vi "Flame Detect Debug.vi"() -> ()   [LabVIEW 2013]
panel:
  in  "Board":enum16{"Rows 1-8", "Rows 9-17", "Rows 18-24"}(ring)
  out "Waveform Chart":T1(graph)
  in  "stop":bool
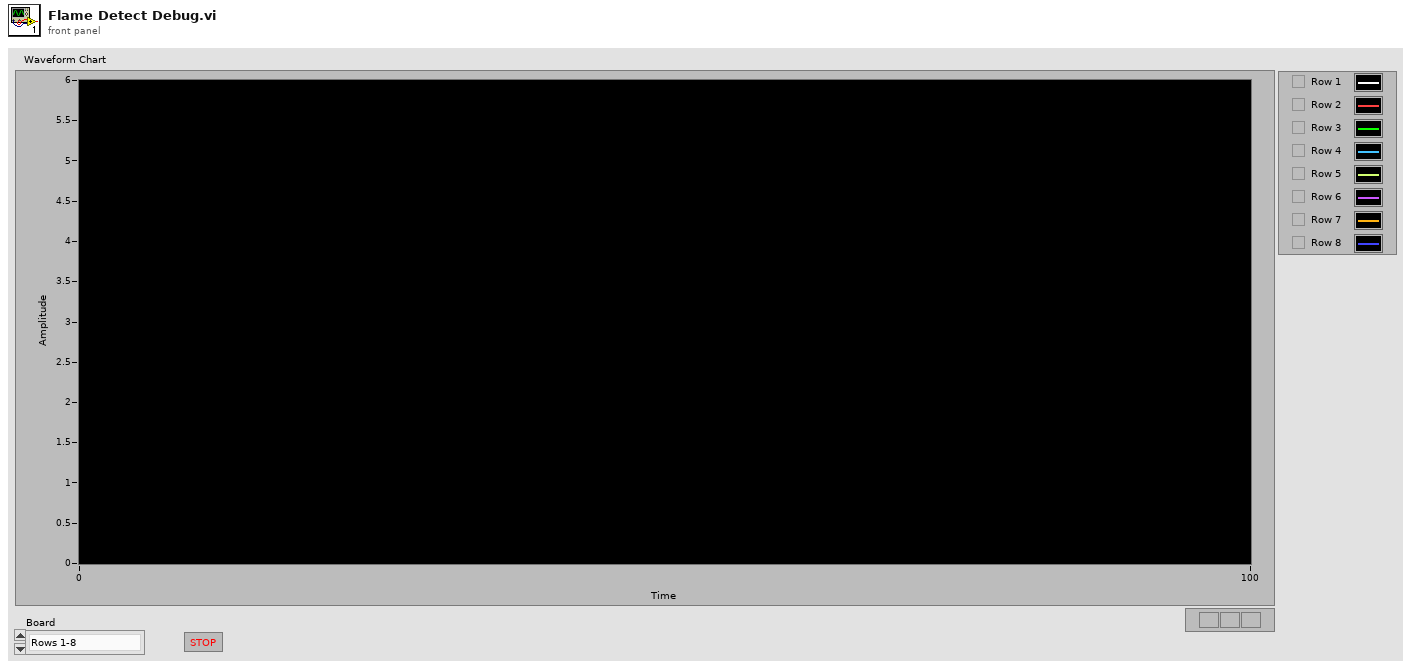
[diagram p1: front panel]
types:
  T1 = cluster{"[0]":dbl, "[1]":dbl, "[2]":dbl, "[3]":dbl, "[4]":dbl, "[5]":dbl, "[6]":dbl, "[7]":dbl, "[8]":dbl}
  T2 = enum16{"HSCAN", "MSCAN", "SWCAN", "LSFTCAN", "HSCAN2", "HSCAN3"}
  T3 = cluster{"DeviceType":i32, "Handle":i32, "NumberOfClients":i32, "SerialNumber":i32, "MaxAllowedClients":i32}[]
  T4 = cluster{"DeviceType":i32, "Handle":i32, "NumberOfClients":i32, "SerialNumber":i32, "MaxAllowedClients":i32}
  T5 = typedef "ctl spymessage.ctl" = cluster{"StatusBitField":u32, "StatusBitField2":u32, "TimeHardware":u32, "TimeHardware2":u32, "TimeSystem":u32, "TimeSystem2":u32, "TimeStampHardwareID":u8, "TimeStampHardwareID2":u8, "NetworkID":u8, "NodeID":u8, "Protocol":u8, "MessagePieceID":u8, "ColorID":u8, "NumberBytesHeader":u8, "NumberBytesData":u8, "DescriptionID":u16, "ArbIDOrHeader":u32, "Data [8]":u8[], "AckBytes [8]":u8[], "Value":sgl, "MiscData":u8}
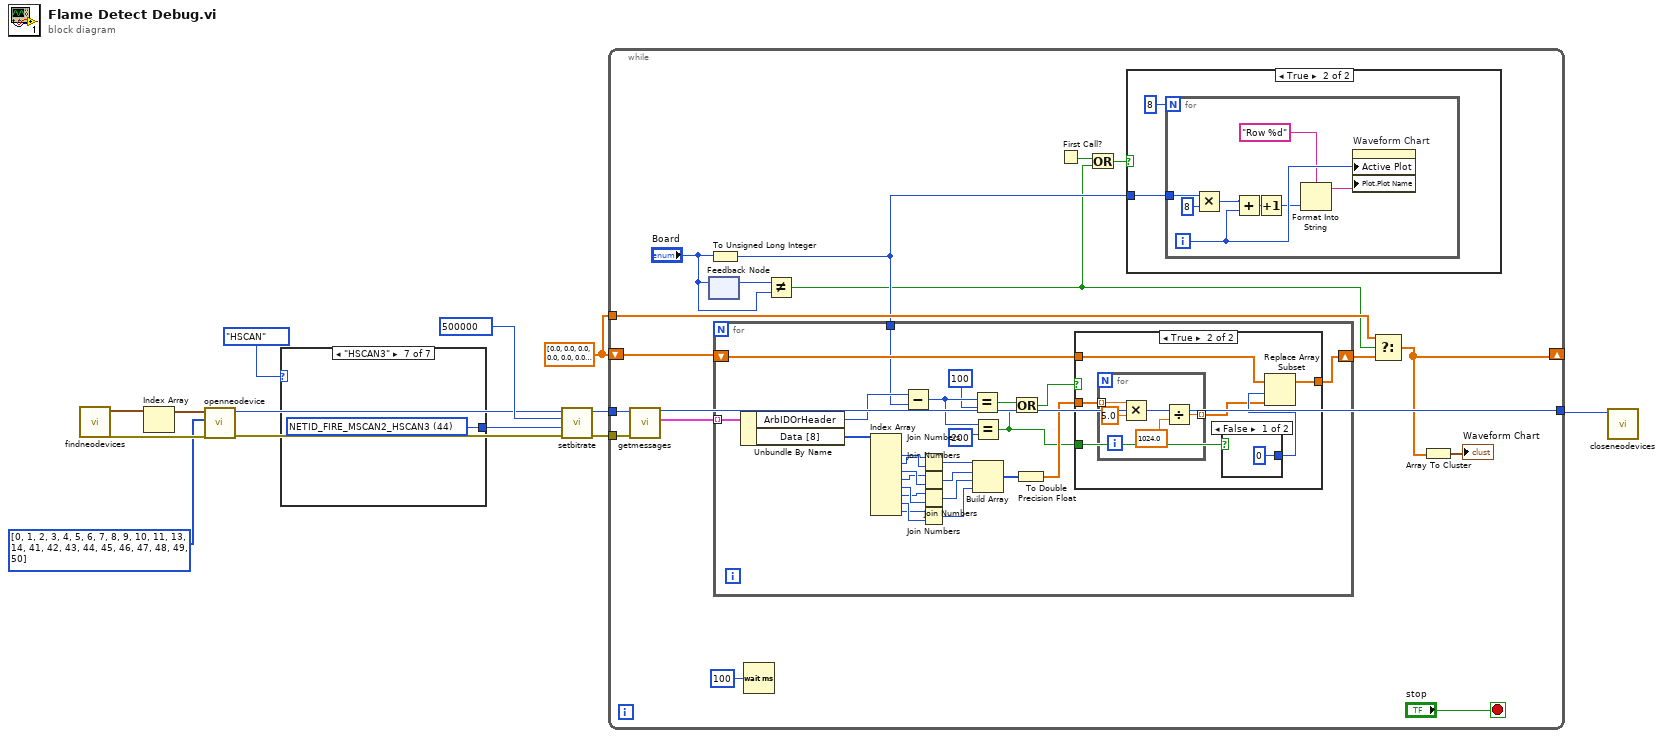
[diagram p0: block diagram]
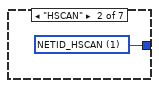
[diagram p3: hidden frame]
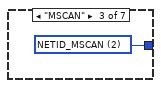
[diagram p4: hidden frame]
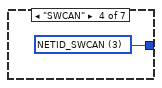
[diagram p5: hidden frame]
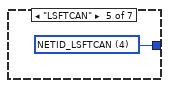
[diagram p6: hidden frame]
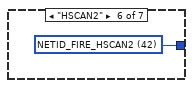
[diagram p7: hidden frame]
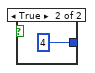
[diagram p10: hidden frame]
diagram:
  w7 = 500000 items=["20000"=20000, "33333"=33333, "50000"=50000, "62500"=62500, "83333"=83333, "100000"=100000, "125000"=125000, "250000"=250000, "500000"=500000, "800000"=800000, "1000000"=1000000] ("Bit Rate")
  w1 = dbl[] [0.0, 0.0, 0.0, 0.0, 0.0, 0.0, 0.0, 0.0]
  w10 = i8[] [0, 1, 2, 3, 4, 5, 6, 7, 8, 9, 10, 11, 13, 14, 41, 42, 43, 44, 45, 46, 47, 48, 49, 50] items=["NETID_DEVICE"=0, "NETID_HSCAN"=1, "NETID_MSCAN"=2, "NETID_SWCAN"=3, "NETID_LSFTCAN"=4, "NETID_FORDSCP"=5, "NETID_J1708"=6, "NETID_AUX"=7, "NETID_JVPW"=8, "NETID_ISO_LIN"=9, "NETID_ISOPIC"=10, "NETID_MAIN51"=11, "NETID_SCI"=13, "NETID_ISO2"=14, "NETID_FIRE_HSCAN1"=41, "NETID_FIRE_HSCAN2"=42, "NETID_FIRE_MSCAN1"=43, "NETID_FIRE_MSCAN2_HSCAN3"=44, "NETID_FIRE_SWCAN"=45, "NETID_FIRE_LSFT"=46, "NETID_FIRE_LIN1"=47, "NETID_FIRE_LIN2"=48, "NETID_FIRE_LIN3"=49, "NETID_FIRE_LIN4"=50] ("bNetworkIDs")
  n1 = call "findneodevices.vi"() -> ("error out"=w12:errorcluster, "NeoDevices {}"=w13:T3)  [unwired: 3 in, 7 out]
  n2 = Index Array(array=w13) -> (element=w11:T4)  [unwired: 1 in]
  n3 = call "openneodevice.vi"("error in (no error)"=w12, "bNetworkIDs"=w10, "NeoDevice{}"=w11) -> ("error out"=w4:errorcluster, "hObject"=w5:i32)  [unwired: 2 in, 5 out]
  n4 = case shown="\"HSCAN3\"" T2."HSCAN" ("CAN Channel") {
    tunnel: [_ w14 w15 w16 w17 w18 w19] -> w6
    frame Default {
    }
    frame "HSCAN" {
      w14 = i8 1 items=["NETID_DEVICE"=0, "NETID_HSCAN"=1, "NETID_MSCAN"=2, "NETID_SWCAN"=3, "NETID_LSFTCAN"=4, "NETID_FORDSCP"=5, "NETID_J1708"=6, "NETID_AUX"=7, "NETID_JVPW"=8, "NETID_ISO_LIN"=9, "NETID_ISOPIC"=10, "NETID_MAIN51"=11, "NETID_SCI"=13, "NETID_ISO2"=14, "NETID_FIRE_HSCAN1"=41, "NETID_FIRE_HSCAN2"=42, "NETID_FIRE_MSCAN1"=43, "NETID_FIRE_MSCAN2_HSCAN3"=44, "NETID_FIRE_SWCAN"=45, "NETID_FIRE_LSFT"=46, "NETID_FIRE_LIN1"=47, "NETID_FIRE_LIN2"=48, "NETID_FIRE_LIN3"=49, "NETID_FIRE_LIN4"=50] ("NetworkID")
    }
    frame "MSCAN" {
      w15 = i8 2 items=["NETID_DEVICE"=0, "NETID_HSCAN"=1, "NETID_MSCAN"=2, "NETID_SWCAN"=3, "NETID_LSFTCAN"=4, "NETID_FORDSCP"=5, "NETID_J1708"=6, "NETID_AUX"=7, "NETID_JVPW"=8, "NETID_ISO_LIN"=9, "NETID_ISOPIC"=10, "NETID_MAIN51"=11, "NETID_SCI"=13, "NETID_ISO2"=14, "NETID_FIRE_HSCAN1"=41, "NETID_FIRE_HSCAN2"=42, "NETID_FIRE_MSCAN1"=43, "NETID_FIRE_MSCAN2_HSCAN3"=44, "NETID_FIRE_SWCAN"=45, "NETID_FIRE_LSFT"=46, "NETID_FIRE_LIN1"=47, "NETID_FIRE_LIN2"=48, "NETID_FIRE_LIN3"=49, "NETID_FIRE_LIN4"=50] ("NetworkID")
    }
    frame "SWCAN" {
      w16 = i8 3 items=["NETID_DEVICE"=0, "NETID_HSCAN"=1, "NETID_MSCAN"=2, "NETID_SWCAN"=3, "NETID_LSFTCAN"=4, "NETID_FORDSCP"=5, "NETID_J1708"=6, "NETID_AUX"=7, "NETID_JVPW"=8, "NETID_ISO_LIN"=9, "NETID_ISOPIC"=10, "NETID_MAIN51"=11, "NETID_SCI"=13, "NETID_ISO2"=14, "NETID_FIRE_HSCAN1"=41, "NETID_FIRE_HSCAN2"=42, "NETID_FIRE_MSCAN1"=43, "NETID_FIRE_MSCAN2_HSCAN3"=44, "NETID_FIRE_SWCAN"=45, "NETID_FIRE_LSFT"=46, "NETID_FIRE_LIN1"=47, "NETID_FIRE_LIN2"=48, "NETID_FIRE_LIN3"=49, "NETID_FIRE_LIN4"=50] ("NetworkID")
    }
    frame "LSFTCAN" {
      w17 = i8 4 items=["NETID_DEVICE"=0, "NETID_HSCAN"=1, "NETID_MSCAN"=2, "NETID_SWCAN"=3, "NETID_LSFTCAN"=4, "NETID_FORDSCP"=5, "NETID_J1708"=6, "NETID_AUX"=7, "NETID_JVPW"=8, "NETID_ISO_LIN"=9, "NETID_ISOPIC"=10, "NETID_MAIN51"=11, "NETID_SCI"=13, "NETID_ISO2"=14, "NETID_FIRE_HSCAN1"=41, "NETID_FIRE_HSCAN2"=42, "NETID_FIRE_MSCAN1"=43, "NETID_FIRE_MSCAN2_HSCAN3"=44, "NETID_FIRE_SWCAN"=45, "NETID_FIRE_LSFT"=46, "NETID_FIRE_LIN1"=47, "NETID_FIRE_LIN2"=48, "NETID_FIRE_LIN3"=49, "NETID_FIRE_LIN4"=50] ("NetworkID")
    }
    frame "HSCAN2" {
      w18 = i8 42 items=["NETID_DEVICE"=0, "NETID_HSCAN"=1, "NETID_MSCAN"=2, "NETID_SWCAN"=3, "NETID_LSFTCAN"=4, "NETID_FORDSCP"=5, "NETID_J1708"=6, "NETID_AUX"=7, "NETID_JVPW"=8, "NETID_ISO_LIN"=9, "NETID_ISOPIC"=10, "NETID_MAIN51"=11, "NETID_SCI"=13, "NETID_ISO2"=14, "NETID_FIRE_HSCAN1"=41, "NETID_FIRE_HSCAN2"=42, "NETID_FIRE_MSCAN1"=43, "NETID_FIRE_MSCAN2_HSCAN3"=44, "NETID_FIRE_SWCAN"=45, "NETID_FIRE_LSFT"=46, "NETID_FIRE_LIN1"=47, "NETID_FIRE_LIN2"=48, "NETID_FIRE_LIN3"=49, "NETID_FIRE_LIN4"=50] ("NetworkID")
    }
    frame "HSCAN3" {
      w19 = i8 44 items=["NETID_DEVICE"=0, "NETID_HSCAN"=1, "NETID_MSCAN"=2, "NETID_SWCAN"=3, "NETID_LSFTCAN"=4, "NETID_FORDSCP"=5, "NETID_J1708"=6, "NETID_AUX"=7, "NETID_JVPW"=8, "NETID_ISO_LIN"=9, "NETID_ISOPIC"=10, "NETID_MAIN51"=11, "NETID_SCI"=13, "NETID_ISO2"=14, "NETID_FIRE_HSCAN1"=41, "NETID_FIRE_HSCAN2"=42, "NETID_FIRE_MSCAN1"=43, "NETID_FIRE_MSCAN2_HSCAN3"=44, "NETID_FIRE_SWCAN"=45, "NETID_FIRE_LSFT"=46, "NETID_FIRE_LIN1"=47, "NETID_FIRE_LIN2"=48, "NETID_FIRE_LIN3"=49, "NETID_FIRE_LIN4"=50] ("NetworkID")
    }
  }
  n5 = call "setbitrate.vi"("error in (no error)"=w4, "NetworkID"=w6, "BitRate"=w7, "hObject"=w5) -> ("error out"=w2:errorcluster, "hObject Out"=w3:i32)  [unwired: 6 out]
  n6 = while {
    tunnel: w3 -> [w35]
    tunnel: w2 -> [w34]
    tunnel: [w31] -> w9
    shift-right: [w25] -> _
    shift-left: w1 -> [w30]
    tunnel: w1 -> [w24]
    stop <- "stop" stop-if-true
    n7 = call "getmessages.vi"("error in (no error)"=w34, "hObject"=w35) -> ("pMsgs"=w36:T5[], "hObject Out"=w31:i32)  [unwired: 8 out]
    n8 = feedback-in #1("Board") -> ()
    n9 = feedback #1() -> (w28:enum16{"Rows 1-8", "Rows 9-17", "Rows 18-24"})  [unwired: 1 in]
    n10 = To Unsigned Long Integer(number="Board") -> (unsigned 32bit integer=w23:u32)
    n11 = for {
      tunnel: w36 -> [w72] mode=indexing
      shift-right: [w47] -> w26
      shift-left: w30 -> [w58]
      tunnel: w23 -> [w54]
      n12 = Unbundle By Name(w72) -> ("ArbIDOrHeader"=w55:u32, "Data [8]"=w71:u8[])
      n13 = Index Array(array=w71) -> (element #1=w70:u8, element #2=w69:u8, element #3=w68:u8, element #4=w67:u8, element #5=w66:u8, element #6=w65:u8, element #7=w64:u8, element #8=w63:u8)  [unwired: 8 in]
      n14 = Subtract(x=w55, y=w54) -> (x-y=w53:u32)
      n15 = Join Numbers(hi=w69, lo=w70) -> ((hi.lo)=w62:u16)
      n16 = Join Numbers(hi=w67, lo=w68) -> ((hi.lo)=w61:u16)
      n17 = Join Numbers(hi=w65, lo=w66) -> ((hi.lo)=w60:u16)
      n18 = Join Numbers(hi=w63, lo=w64) -> ((hi.lo)=w59:u16)
      n19 = Equal?(x=w53, y=u32 100) -> (x = y?=w50:bool)
      n20 = Equal?(x=w53, y=u32 200) -> (x = y?=w48:bool)
      n21 = Build Array(w62, w61, w60, w59) -> (w57:u16[])
      n22 = Or(x=w50, y=w48) -> (x .or. y?=w49:bool)
      n23 = To Double Precision Float(number=w57) -> (double precision float=w56:dbl[])
      n24 = case shown="True" w49 {
        tunnel: w58 -> [w73 w79]
        tunnel: w56 -> [_ w75]
        tunnel: [w73 w76] -> w47
        tunnel: w48 -> [_ w78]
        frame False {
        }
        frame True {
          n25 = for {
            tunnel: w75 -> [w81] mode=indexing
            tunnel: [w80] -> w74 mode=indexing
            n26 = Multiply(x=w81, y=5.0) -> (x*y=w83:dbl)
            n27 = Divide(x=w83, y=1024.0) -> (x/y=w80:dbl)
          }
          n28 = case shown="False" w78 {
            tunnel: [0 ("index") 4 ("index")] -> w77
            frame False {
            }
            frame True {
            }
          }
          n29 = Replace Array Subset(array=w79, new element=w74, index=w77) -> (w76:dbl[])
        }
      }
    }
    n30 = Wait (ms)(milliseconds to wait=u32 100) -> ()  [unwired: 1 out]
    n31 = Not Equal?(x=w28, y="Board") -> (x != y?=w21:bool)
    n32 = First Call?() -> (First Call?: T/F=w22:bool)
    n33 = Or(x=w22, y=w21) -> (x .or. y?=w20:bool)
    n34 = case shown="True" w20 {
      tunnel: w23 -> [_ w37]
      frame False {
      }
      frame True {
        n35 = for {
          N: 8 -> [_]
          tunnel: w37 -> [w46]
          i -> [w43]
          n36 = Multiply(x=w46, y=u32 8) -> (x*y=w44:u32)
          n37 = Add(x=w44, y=w43) -> (x+y=w42:u32)
          n38 = Increment(x=w42) -> (x+1=w39:u32)
          n39 = Format Into String(format string="Row %d", w39) -> (resulting string=w40:string)  [unwired: 2 in, 1 out]
          n40 = property on="Waveform Chart" class="WFChart (strict)"("Active Plot"=w43, "Plot.Plot Name"=w40) -> ()  [unwired: 2 in, 2 out]
        }
      }
    }
    n41 = Select(t=w24, s=w21, f=w26) -> (s? t:f=w25:dbl[])
    n42 = Array To Cluster(array=w25) -> (cluster=→"Waveform Chart":T1)
  }
  n43 = call "closeneodevices.vi"("hObject"=w9) -> ()  [unwired: 2 in, 9 out]
